vi "Splite MultiLine Cell.vi"(8 "error in (no error)":errorcluster, 10 "Col Index":i32, 11 "CfgTable in":string[][](array[string])) -> (0 "error out":errorcluster, 3 "CfgTable out":string[][](array[string]))   [LabVIEW 2017, in "ClusterCfgTable.lvlib"]
uses:
  ClusterCfgTable.lvlib
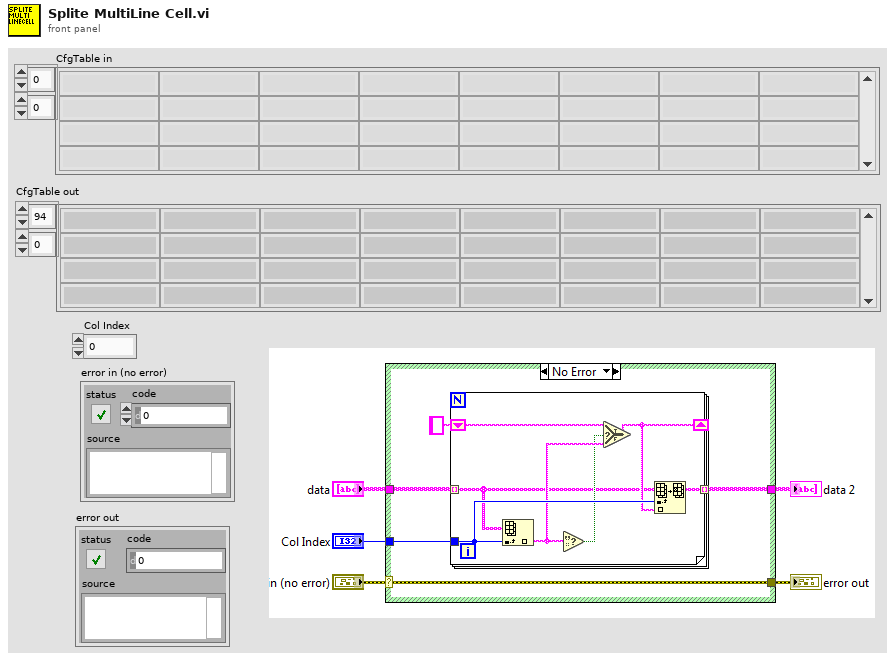
[diagram p1: front panel]
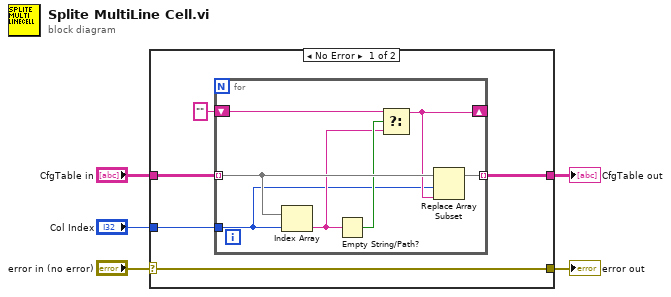
[diagram p0: block diagram]
diagram:
  n1 = case shown="No Error" "error in (no error)" {
    selector: "error in (no error)" -> [w10 w19]
    tunnel: [w10 w19] -> w5
    tunnel: "Col Index" -> [w9 _]
    tunnel: [w8 w18] -> w2
    tunnel: "CfgTable in" -> [w7 w18]
    frame No Error {
      n2 = for {
        tunnel: w7 -> [w17] mode=indexing
        tunnel: [w13] -> w8 mode=indexing
        shift-right: [w12] -> _
        shift-left: "" ("element") -> [w14]
        tunnel: w9 -> [w11]
        n3 = Index Array(array=w17, index=w11) -> (element=w15:string)
        n4 = Empty String/Path?(string/path=w15) -> (empty?=w16:bool)
        n5 = Select(t=w14, s=w16, f=w15) -> (s? t:f=w12:string)
        n6 = Replace Array Subset(array=w17, new element=w12, index=w11) -> (w13:string[])
      }
    }
    frame Error {
    }
  }
  "error out" <- w5
  "CfgTable out" <- w2
